vi "LV86_SelectROI.vi"(3 "Image":T2 {"Dialogs" format="%.0b"}) -> (0 "Rect":T1, 1 "Image":T2 {"Dialogs" format="%.0b"})   [LabVIEW 2024]
doc: "This VI pops up a window where the user can select a region of interest."
uses:
  <userlib>/ImageProcessing/QTLIB_2595_LV86/QT_Image.ctl
panel:
  in  "Pen":u32(colorbox)=16777217
  in  "ROI":T1
  out "Image":picture
  in  "OK":bool
  out "Display":picture caption="new picture"
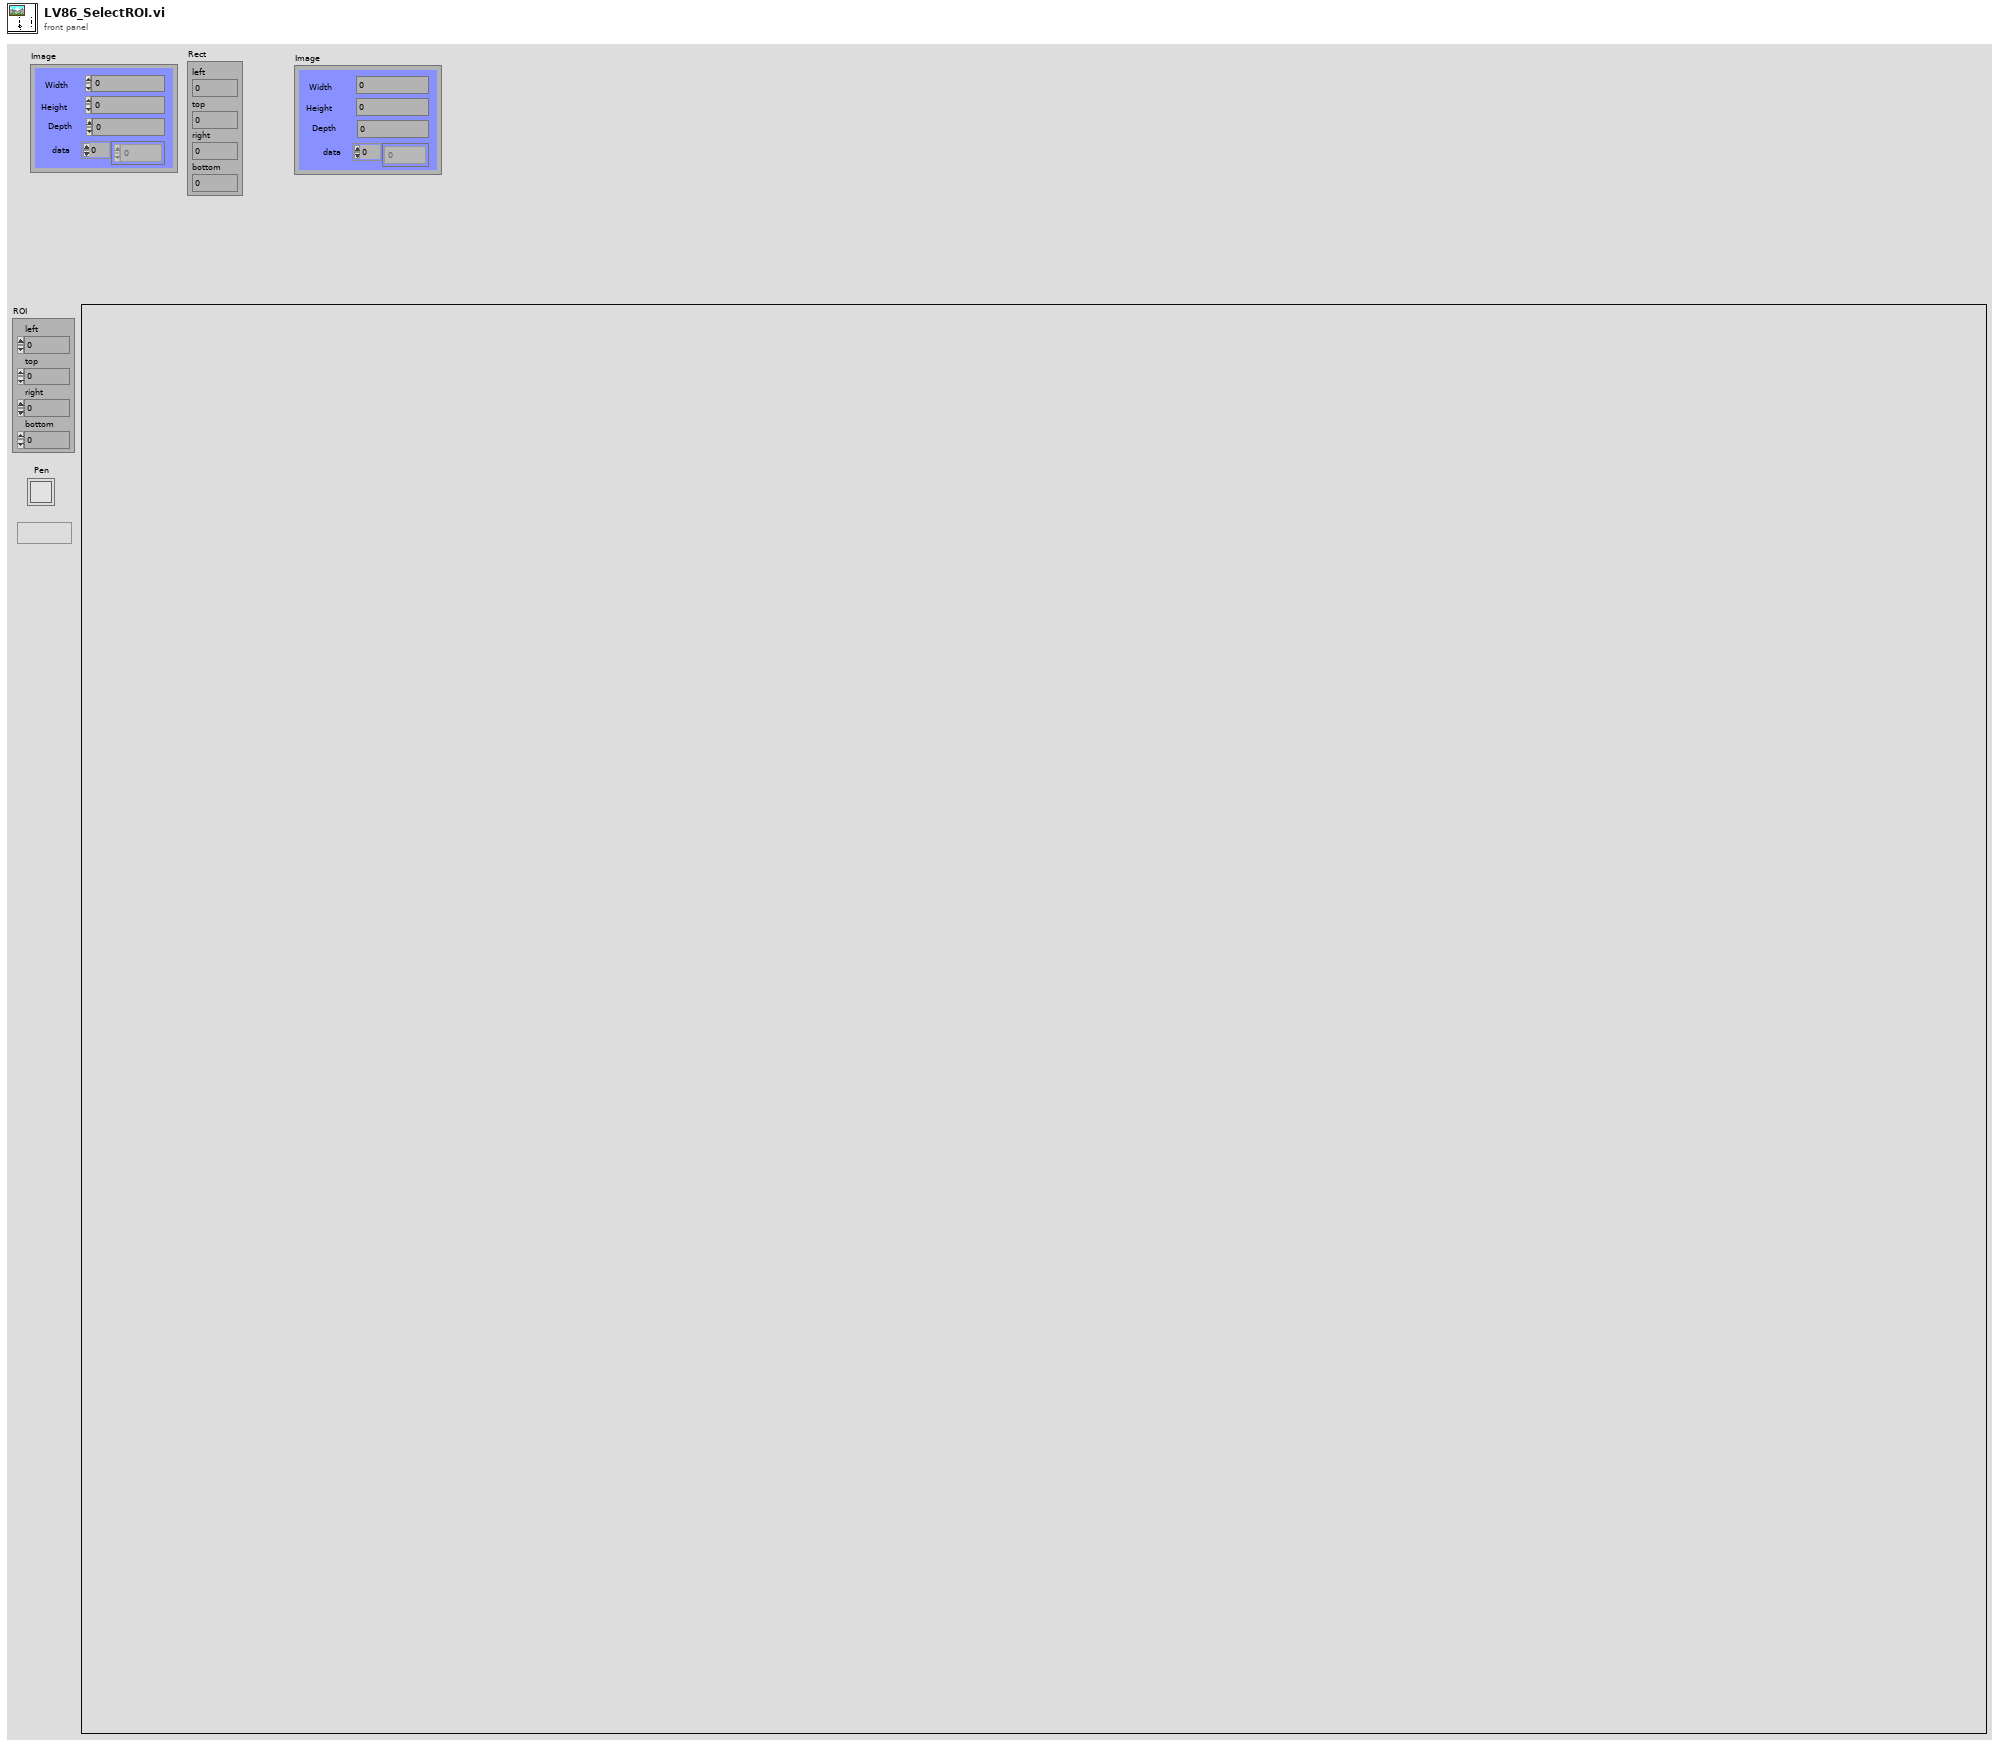
[diagram p1: front panel]
types:
  T1 = cluster{"left":i32, "top":i32, "right":i32, "bottom":i32}
  T2 = typedef "QT_Image.ctl" = cluster{"Width":i32, "Height":i32, "Depth":i32, "data":u8[], "Compressed data":u8[], "Color table":u32[], "Duration":i32, "Options":i32, "Timestamp":i32, "ID":i32, "Reserved":i32, "Dialogs":u32}
  T3 = typedef "LVRectTypeDef.ctl" = cluster{"left":i16, "top":i16, "right":i16, "bottom":i16}
  T4 = typedef "LVMouseTypeDef.ctl" = cluster{"Mouse Position":cluster{"X":i32, "Y":i32}, "Mouse Modifiers":cluster{"Button Down":bool, "Shift Mod":bool, "Menu Mod":bool, "Option Mod":bool}}
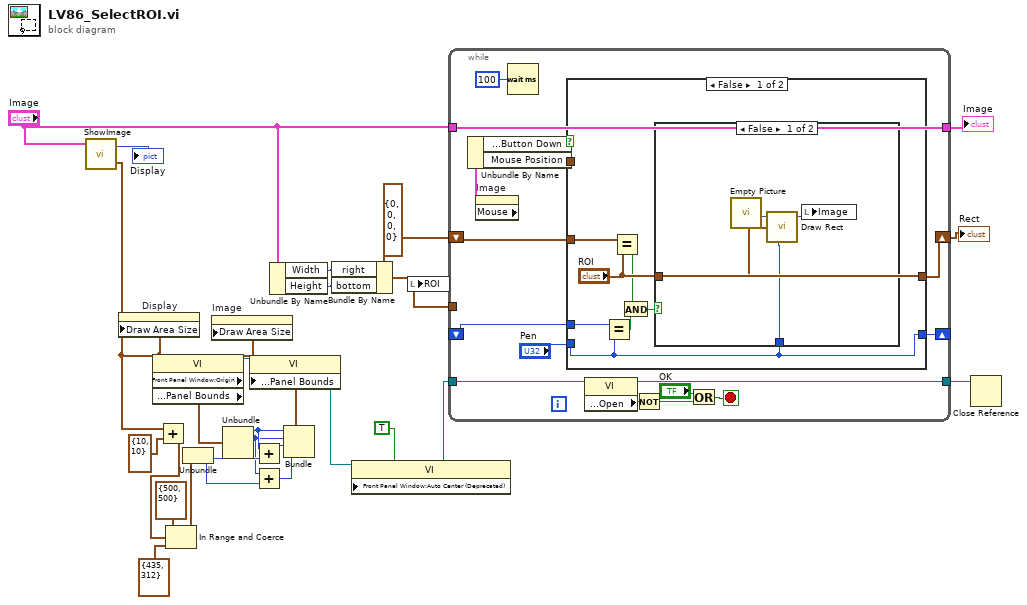
[diagram p0: block diagram]
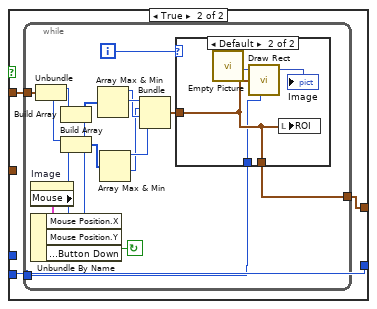
[diagram p3: hidden frame]
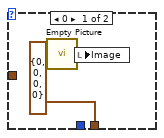
[diagram p4: hidden frame]
diagram:
  w7 = T1 {"left"=0, "top"=0, "right"=0, "bottom"=0} ("ROI")
  n1 = call <userlib>:"ShowImage.vi"("Image"="Image") -> ("dimensions"=w2:cluster{"Witdh":i32, "Height":i32}, "image"=→"Display":picture)  [unwired: 2 in]
  n2 = property on="Display" class="Pict"("Draw Area Size"=w2) -> ()  [unwired: 2 in, 2 out]
  n3 = property class="VI" props=["Front Panel Window:Origin", "Front Panel Window:Panel Bounds"]() -> (reference out=w24:refnum<vi>, "Front Panel Window:Panel Bounds"=w18:T3)  [unwired: 2 in, 2 out]
  n4 = Add(x=w2, y=cluster{i32, i32} {10, 10} ("x+y")) -> (x+y=w9:cluster{i32, i32})
  n5 = In Range and Coerce(upper limit=cluster{i32, i32} {500, 500}, x=w9, lower limit=cluster{i32, i32} {435, 312} ("x+y")) -> (coerced(x)=w8:cluster{i32, i32})  [unwired: 1 out]
  n6 = Unbundle(w8) -> (w15:i32, w14:i32)
  n7 = property on="Image" class="Pict"("Draw Area Size"=w2) -> ()  [unwired: 2 in, 2 out]
  n8 = Unbundle(w18) -> ("left"=w13:i16, "top"=w12:i16)  [unwired: 2 out]
  n9 = Add(x=w13, y=w15) -> (x+y=w17:i32)
  n10 = Add(x=w12, y=w14) -> (x+y=w16:i32)
  n11 = Unbundle By Name("Image") -> ("Width"=w6:i32, "Height"=w5:i32)
  n12 = Bundle("left"=w13, "top"=w12, w17, w16) -> (w22:cluster{"left":i16, "top":i16, i32, i32})  [unwired: 1 out]
  n13 = property class="VI"(reference=w24, "Front Panel Window:Panel Bounds"=w22) -> (reference out=w20:refnum<vi>)  [unwired: 1 in, 1 out]
  n14 = Bundle By Name(cluster=w7, "right"=w6, "bottom"=w5) -> (w4:T1)
  n15 = property class="VI"(reference=w20, "Front Panel Window:Auto Center (Deprecated)"=TRUE ("Front Panel Window:Auto Center")) -> (reference out=w21:refnum<vi>)  [unwired: 1 in, 1 out]
  n16 = local write "ROI"(w4) -> ()
  n17 = while {
    shift-left: _ -> [w28]
    shift-right: [w30] -> _
    tunnel: w4 -> [_]
    shift-left: w7 -> [w32]
    shift-right: [w33] -> w25
    tunnel: [w29] -> w26
    tunnel: w21 -> [w39]
    tunnel: [w41] -> w27
    tunnel: "Image" -> [w41]
    stop <- w35 stop-if-true
    n18 = property on="Image" class="Pict"() -> ("Mouse"=w43:T4)  [unwired: 2 in, 2 out]
    n19 = Unbundle By Name(w43) -> ("Mouse Modifiers.Button Down"=w34:bool, "Mouse Position"=w42:cluster{"X":i32, "Y":i32})
    n20 = Wait (ms)(milliseconds to wait=u32 100) -> ()  [unwired: 1 out]
    n21 = case shown="False" w34 {
      tunnel: w42 -> [_ w57]
      tunnel: ["ROI" w56] -> w33
      tunnel: w32 -> [w50 _]
      tunnel: "Pen" -> [w47 w55]
      tunnel: [w47 w55] -> w30
      tunnel: w28 -> [w48 _]
      frame False {
        n22 = Equal?(x=w48, y=w47) -> (x = y?=w46:bool)
        n23 = Equal?(x=w50, y="ROI") -> (x = y?=w45:bool)
        n24 = And(x=w45, y=w46) -> (x .and. y?=w44:bool)
        n25 = case shown="False" w44 {
          tunnel: "ROI" -> [w52 _]
          tunnel: w47 -> [w51 _]
          frame False {
            n26 = call "Empty Picture"() -> ("empty picture"=w54:picture)
            n27 = call <vilib>:"Draw Rect.vi"("picture"=w54, "rect"=w52, "color(black)"=w51) -> ("new picture"=w53:picture)  [unwired: 2 in, 4 out]
            n28 = local write "Image"(w53) -> ()
          }
          frame True {
          }
        }
      }
      frame True {
        n29 = while {
          tunnel: w55 -> [w58]
          tunnel: [w59] -> w56
          tunnel: w57 -> [w71]
          i -> [w74]
          stop <- w72 continue-if-true
          n30 = property on="Image" class="Pict"() -> ("Mouse"=w73:T4)  [unwired: 2 in, 2 out]
          n31 = Unbundle By Name(w73) -> ("Mouse Position.X"=w69:i32, "Mouse Position.Y"=w67:i32, "Mouse Modifiers.Button Down"=w72:bool)
          n32 = Unbundle(w71) -> ("X"=w70:i32, "Y"=w68:i32)
          n33 = Build Array(w70, w69) -> (w66:i32[])
          n34 = Build Array(w68, w67) -> (w63:i32[])
          n35 = Array Max & Min(array=w66) -> (max value=w64:i32, min value=w65:i32)  [unwired: 2 out]
          n36 = Array Max & Min(array=w63) -> (max value=w62:i32, min value=w61:i32)  [unwired: 2 out]
          n37 = Bundle(w65, w61, w64, w62) -> (w60:cluster{i32, i32, i32, i32})  [unwired: 1 out]
          n38 = case shown="Default" w74 {
            tunnel: w60 -> [_ w80]
            tunnel: [cluster{i32, i32, i32, i32} {0, 0, 0, 0} w80] -> w59
            tunnel: w58 -> [_ w77]
            frame 0 {
              n39 = call "Empty Picture"() -> ("empty picture"=w76:picture)
              n40 = local write "Image"(w76) -> ()
            }
            frame Default {
              n41 = call "Empty Picture"() -> ("empty picture"=w79:picture)
              n42 = call <vilib>:"Draw Rect.vi"("picture"=w79, "rect"=w80, "color(black)"=w77) -> ("new picture"=→"Image":picture)  [unwired: 2 in, 4 out]
              n43 = local write "ROI"(w80) -> ()
            }
          }
        }
      }
    }
    n44 = property class="VI"(reference=w39) -> (reference out=w29:refnum<vi>, "Front Panel Window:Open"=w38:bool)  [unwired: 1 in, 1 out]
    n45 = Not(x=w38) -> (.not. x?=w36:bool)
    n46 = Or(x="OK", y=w36) -> (x .or. y?=w35:bool)
  }
  "Image" <- w27
  "Rect" <- w25
  n47 = Close Reference(reference=w26) -> ()  [unwired: 1 in, 1 out]
